vi "pb_init.vi"(1 "error in (no error)":errorcluster) -> (0 "error out":errorcluster)   [LabVIEW 2013, in "PulseBlaster.lvlib"]
uses:
  PulseBlaster.lvlib
  spinapi.dll
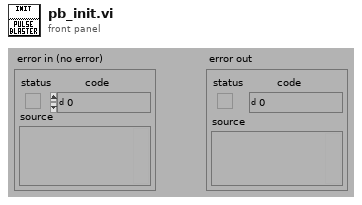
[diagram p1: front panel]
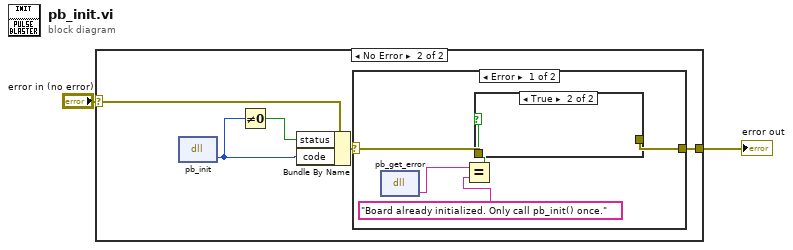
[diagram p0: block diagram]
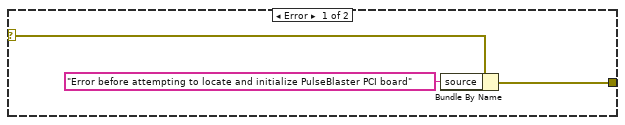
[diagram p2: hidden frame]
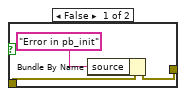
[diagram p3: hidden frame]
diagram:
  n1 = case shown="No Error" "error in (no error)" {
    selector: "error in (no error)" -> [w5 w10]
    tunnel: [w4 w7] -> w1
    frame Error {
      n2 = Bundle By Name(cluster=w5, "source"="Error before attempting to locate and initialize PulseBlaster PCI board") -> (w4:errorcluster)
    }
    frame No Error {
      n3 = dll-call lib="C:/Users/cherold/Documents/SVNrepo_local/branches/TableTest_Auto/codes/DeviceVIs/Pulseblaster/spinapi.dll" fn="pb_init"() -> ("return type"=w6:i32)  [unwired: 3 in, 2 out]
      n4 = Not Equal To 0?(x=w6) -> (x != 0?=w9:bool)
      n5 = Bundle By Name(cluster=w10, "status"=w9, "code"=w6) -> (w8:errorcluster)
      n6 = case shown="Error" w8 {
        selector: w8 -> [w15 w19]
        tunnel: [w14 w19] -> w7
        frame Error {
          n7 = dll-call lib="C:/Users/cherold/Documents/SVNrepo_local/branches/TableTest_Auto/codes/DeviceVIs/Pulseblaster/spinapi.dll" fn="pb_get_error"() -> ("spinerr"=w12:string)  [unwired: 3 in, 2 out]
          n8 = Equal?(x=w12, y="Board already initialized. Only call pb_init() once." ("spinerr")) -> (x = y?=w11:bool)
          n9 = case shown="True" w11 {
            tunnel: w15 -> [w18 _]
            tunnel: [w16 _] -> w14
            frame False {
              n10 = Bundle By Name(cluster=w18, "source"="Error in pb_init") -> (w16:errorcluster)
            }
            frame True {
            }
          }
        }
        frame No Error {
        }
      }
    }
  }
  "error out" <- w1
